vi "test_python_node.vi"() -> ()   [LabVIEW 2025]
panel:
  out "return value":string
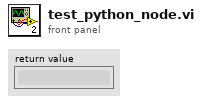
[diagram p1: front panel]
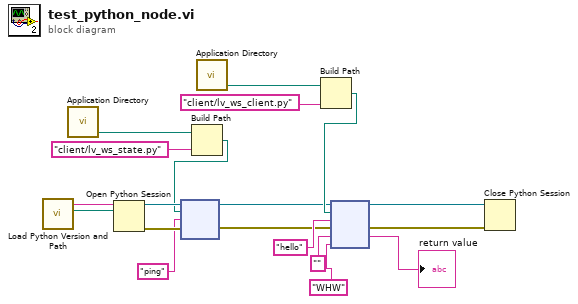
[diagram p0: block diagram]
diagram:
  n1 = call "Load Python Version and Path.vi"() -> ("path"=w13:path, "version"=w14:string)  [unwired: 10 in]
  n2 = call <vilib>:"Application Directory.vi"() -> ("Application Directory"=w3:path)
  n3 = Open Python Session(python version=w14, python path=w13) -> (session out=w8:refnum<k35>, error out=w7:errorcluster)  [unwired: 1 in]
  n4 = Build Path(base path=w3, name or relative path="client/lv_ws_state.py") -> (appended path=w1:path)
  n5 = node(w8, w1, "ping" ("function name"), w7) -> (w5:refnum<k35>, w6:errorcluster)  [unwired: 2 in, 2 out]
  n6 = call <vilib>:"Application Directory.vi"() -> ("Application Directory"=w12:path)
  n7 = Build Path(base path=w12, name or relative path="client/lv_ws_client.py") -> (appended path=w11:path)
  n8 = node(w5, w11, "hello" ("function name"), w6, "", "WHW") -> (w19:refnum<k35>, w18:errorcluster, →"return value":string)  [unwired: 1 in, 2 out]
  n9 = Close Python Session(session in=w19, error in=w18) -> ()  [unwired: 1 out]
